vi "Control Panel.vi"(8 "error in (no error)":errorcluster, 11 "PEM in":refnum<class "PEM.lvclass">) -> (0 "error out":errorcluster, 3 "PEM out":refnum<class "PEM.lvclass">)   [LabVIEW 2017, in "PEM.lvclass"]
doc: "(Dynamic) A user-level application that simulates the physical front panel of the Instrument. Provide the user with buttons to manually control features of the instrument, and provide indicators of its current state."
uses:
  PEM.lvclass
  PEM.lvclass/PEM.ctl
  Utility Classes/Scannable/Scannable.lvclass
panel:
  in  "Set Retardation":dbl=1.0 min=0.0 max=1.0 step=0.001
  out "Curr. Retardation":dbl
  in  "Set Wavelength":dbl[unit] min=0.0 max=1.99999e-05 step=1.0000000000000002e-10
  out "Curr. Wavelength":dbl[unit]
  in  "Inhibit":bool
  out "Ready":bool
  out "Frequency":string
  out "stop":bool
  in  "Set Retardation 2":bool
  in  "Set Wavelength 2":bool
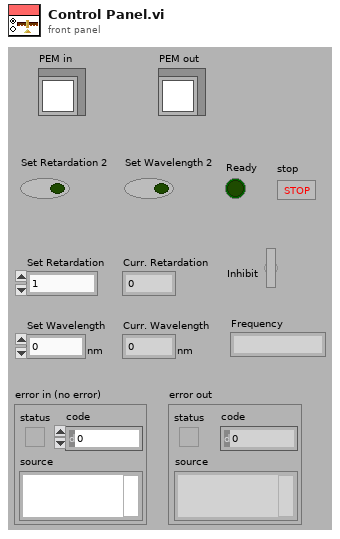
[diagram p1: front panel]
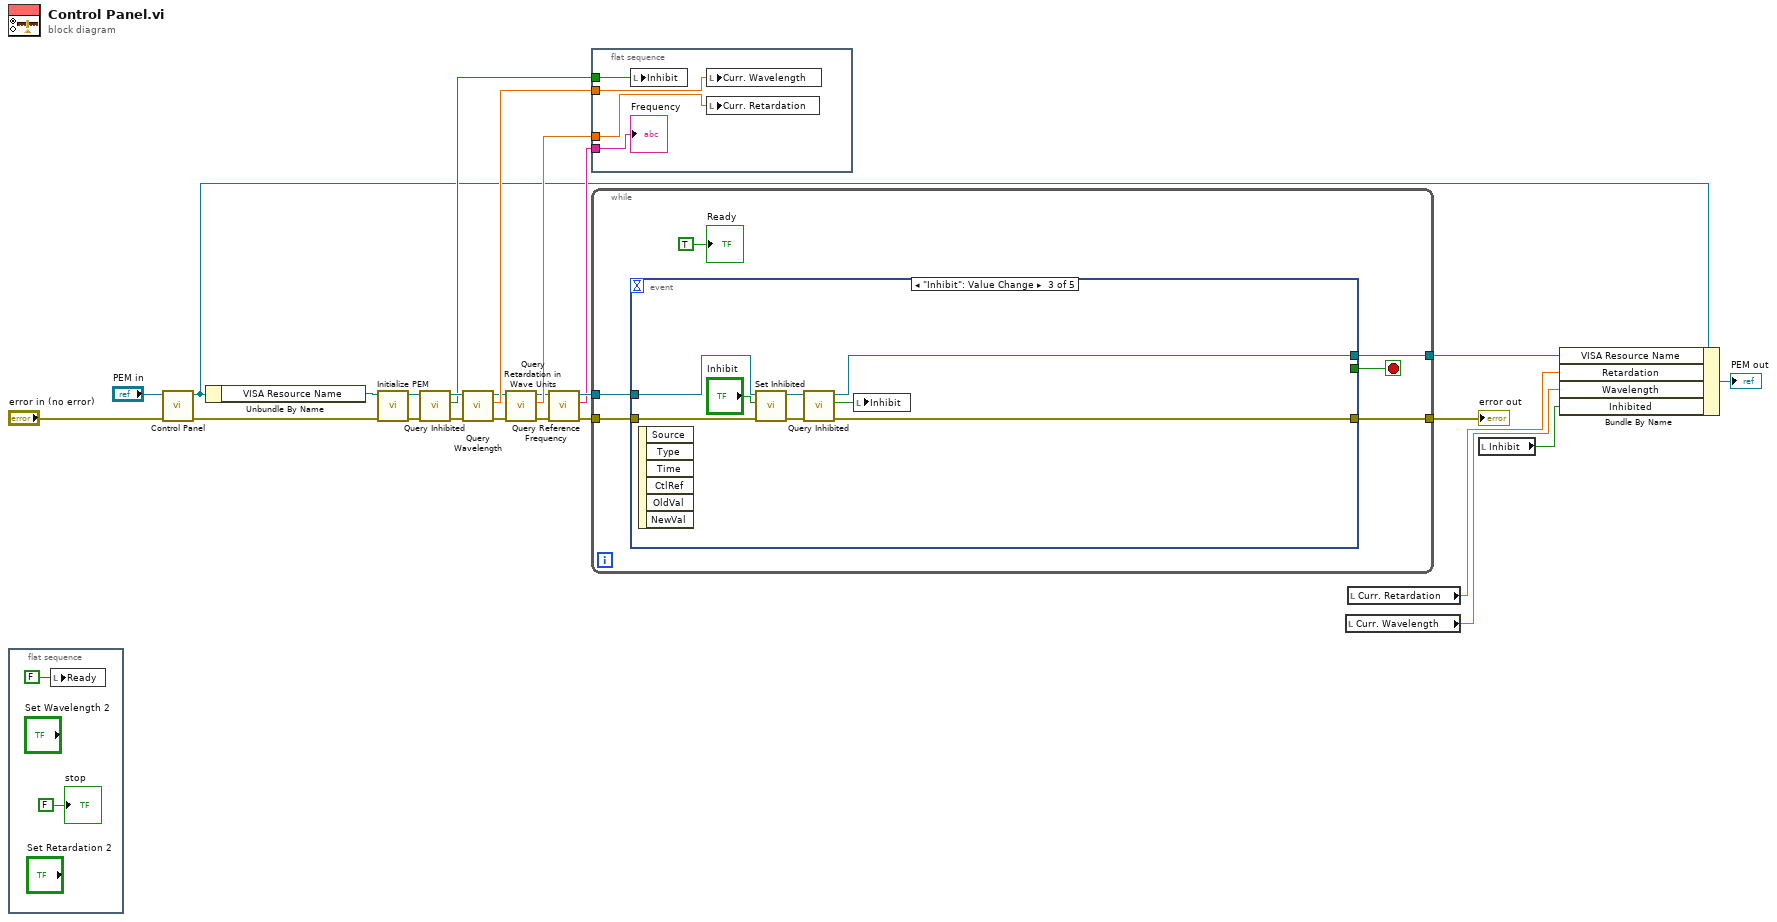
[diagram p0: block diagram]
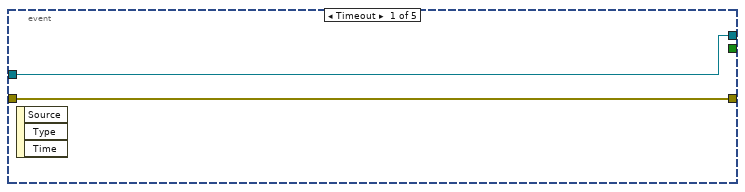
[diagram p2: hidden frame]
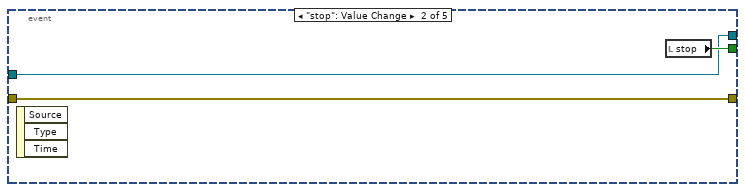
[diagram p3: hidden frame]
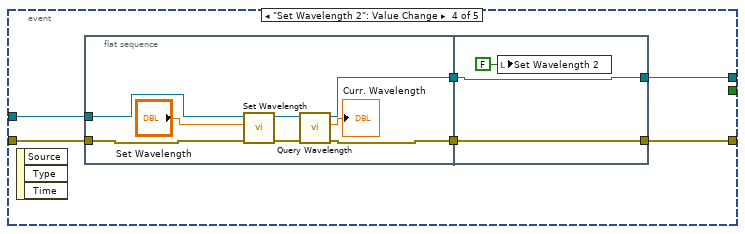
[diagram p4: hidden frame]
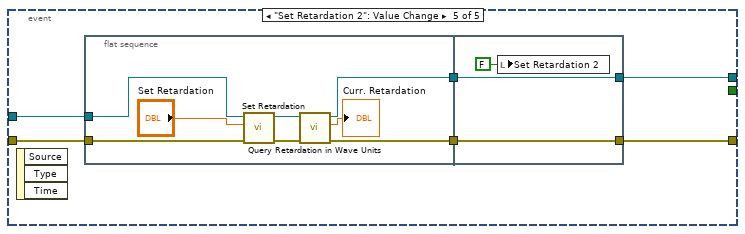
[diagram p5: hidden frame]
diagram:
  n1 = flat-sequence {
    frame #0 {
      n2 = local write "Ready"(FALSE ("Ready")) -> ()
      "stop" <- FALSE ("stop")
    }
  }
  n3 = call-parent "Control Panel.vi"("error in (no error)"="error in (no error)", "Instrument in"="PEM in") -> ("error out"=w9:errorcluster, "Instrument out"=w5:refnum<class "PEM.lvclass">)  [unwired: 8 in]
  n4 = Unbundle By Name(w5) -> ("VISA Resource Name"=w7:refnum<visa-resource-name>)
  n5 = call "Initialize PEM.vi"("error in (no error)"=w9, "VISA resource name"=w7) -> ("error out"=w14:errorcluster, "VISA resource name out"=w13:refnum<visa-resource-name>)  [unwired: 8 in]
  n6 = call "Query Inhibited.vi"("error in (no error)"=w14, "VISA resource name"=w13) -> ("error out"=w11:errorcluster, "Inibit"=w10:bool, "VISA resource name out"=w12:refnum<visa-resource-name>)  [unwired: 7 in]
  n7 = call "Query Wavelength.vi"("error in (no error)"=w11, "VISA resource name"=w12) -> ("error out"=w18:errorcluster, "Wavelength"=w20:dbl[unit], "VISA resource name out"=w17:refnum<visa-resource-name>)  [unwired: 7 in]
  n8 = call "Query Retardation in Wave Units.vi"("error in (no error)"=w18, "VISA resource name"=w17) -> ("error out"=w15:errorcluster, "Fraction of wave Retardation"=w22:dbl, "VISA resource name out"=w16:refnum<visa-resource-name>)  [unwired: 7 in]
  n9 = call "Query Reference Frequency.vi"("error in (no error)"=w15, "VISA resource name"=w16) -> ("error out"=w23:errorcluster, "Frequency output"=w19:string, "VISA resource name out"=w21:refnum<visa-resource-name>)  [unwired: 7 in]
  n10 = flat-sequence {
    tunnel: w22 -> [w31]
    tunnel: w20 -> [w30]
    tunnel: w19 -> [w28]
    tunnel: w10 -> [w29]
    frame #0 {
      n11 = local write "Inhibit"(w29) -> ()
      n12 = local write "Curr. Wavelength"(w30) -> ()
      n13 = local write "Curr. Retardation"(w31) -> ()
      "Frequency" <- w28
    }
  }
  n14 = while {
    tunnel: [w37] -> w8
    tunnel: [w36] -> w4
    tunnel: w23 -> [w34]
    tunnel: w21 -> [w33]
    stop <- w35 stop-if-true
    n15 = event shown="[2] \"Inhibit\": Value Change" {
      selector: _ -> [_ _ _ _ _]
      dyn-events: _ -> [_ _ _ _ _]
      timeout: _ -> [_ _ _ _ _]
      tunnel: w34 -> [w39 w41 w49 w55 w73]
      tunnel: w33 -> [w38 w40 w50 w56 w72]
      tunnel: [w39 w41 w46 w53 w70] -> w37
      tunnel: [w38 w40 w45 w54 w71] -> w36
      tunnel: [_ w42 _ _ _] -> w35
      event Timeout {
        n16 = event-data() -> ()  [unwired: 1 in, 3 out]
      }
      event "stop": Value Change {
        n17 = event-data() -> ()  [unwired: 1 in, 3 out]
        n18 = local read "stop"() -> (w42:bool)
      }
      event "Inhibit": Value Change {
        n19 = event-data() -> ()  [unwired: 1 in, 6 out]
        n20 = call "Set Inhibited.vi"("error in (no error)"=w49, "Inhibit"="Inhibit", "VISA resource name"=w50) -> ("error out"=w47:errorcluster, "VISA resource name out"=w48:refnum<visa-resource-name>)  [unwired: 6 in, 1 out]
        n21 = call "Query Inhibited.vi"("error in (no error)"=w47, "VISA resource name"=w48) -> ("error out"=w46:errorcluster, "Inibit"=w44:bool, "VISA resource name out"=w45:refnum<visa-resource-name>)  [unwired: 7 in]
        n22 = local write "Inhibit"(w44) -> ()
      }
      event "Set Wavelength 2": Value Change {
        n23 = event-data() -> ()  [unwired: 1 in, 3 out]
        n24 = flat-sequence {
          tunnel: w56 -> [w64]
          tunnel: w55 -> [w63]
          tunnel: [w61] -> w52
          tunnel: [w60] -> w51
          tunnel: [w66] -> w53
          tunnel: [w67] -> w54
          tunnel: w52 -> [w67]
          tunnel: w51 -> [w66]
          frame #0 {
            n25 = call "Set Wavelength.vi"("error in (no error)"=w63, "wavelength"="Set Wavelength", "VISA resource name"=w64) -> ("error out"=w58:errorcluster, "VISA resource name out"=w59:refnum<visa-resource-name>)  [unwired: 5 in, 2 out]
            n26 = call "Query Wavelength.vi"("error in (no error)"=w58, "VISA resource name"=w59) -> ("error out"=w60:errorcluster, "Wavelength"=→"Curr. Wavelength":dbl[unit], "VISA resource name out"=w61:refnum<visa-resource-name>)  [unwired: 7 in]
          }
          frame #1 {
            n27 = local write "Set Wavelength 2"(FALSE ("Set Wavelength")) -> ()
          }
        }
      }
      event "Set Retardation 2": Value Change {
        n28 = event-data() -> ()  [unwired: 1 in, 3 out]
        n29 = flat-sequence {
          tunnel: w73 -> [w80]
          tunnel: w72 -> [w79]
          tunnel: [w77] -> w69
          tunnel: [w75] -> w68
          tunnel: [w83] -> w70
          tunnel: [w84] -> w71
          tunnel: w69 -> [w84]
          tunnel: w68 -> [w83]
          frame #0 {
            n30 = call "Set Retardation.vi"("error in (no error)"=w80, "Retardation"="Set Retardation", "VISA resource name"=w79) -> ("error out"=w76:errorcluster, "VISA resource name out"=w78:refnum<visa-resource-name>)  [unwired: 6 in, 1 out]
            n31 = call "Query Retardation in Wave Units.vi"("error in (no error)"=w76, "VISA resource name"=w78) -> ("error out"=w75:errorcluster, "Fraction of wave Retardation"=→"Curr. Retardation":dbl, "VISA resource name out"=w77:refnum<visa-resource-name>)  [unwired: 7 in]
          }
          frame #1 {
            n32 = local write "Set Retardation 2"(FALSE ("Set Retardation")) -> ()
          }
        }
      }
    }
    "Ready" <- TRUE ("Ready")
  }
  "error out" <- w8
  n33 = local read "Curr. Wavelength"() -> (w1:dbl[unit])
  n34 = local read "Curr. Retardation"() -> (w2:dbl)
  n35 = local read "Inhibit"() -> (w3:bool)
  n36 = Bundle By Name(cluster=w5, "VISA Resource Name"=w4, "Retardation"=w2, "Wavelength"=w1, "Inhibited"=w3) -> (→"PEM out":refnum<class "PEM.lvclass">)
